vi "Get EventName.vi"(8 "error in (no error)":errorcluster, 11 "EventData in":refnum<class "EventData.lvclass">) -> (0 "error out":errorcluster, 2 "Event Name":string, 3 "EventData out":refnum<class "EventData.lvclass">)   [LabVIEW 2021, in "EventManagerLibrary.lvlib" / "EventData.lvclass"]
uses:
  EventData.lvclass
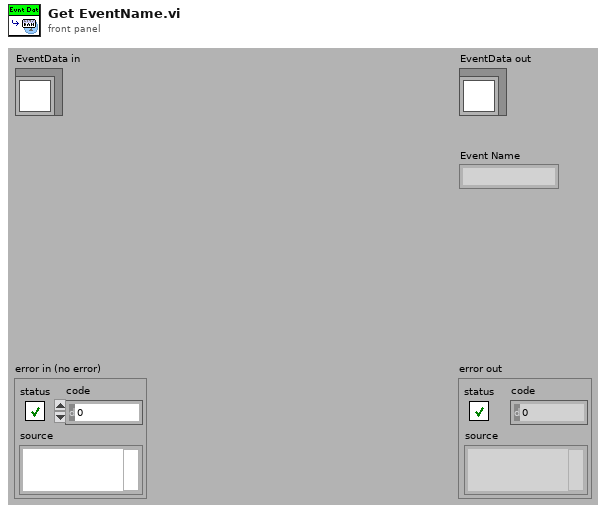
[diagram p1: front panel]
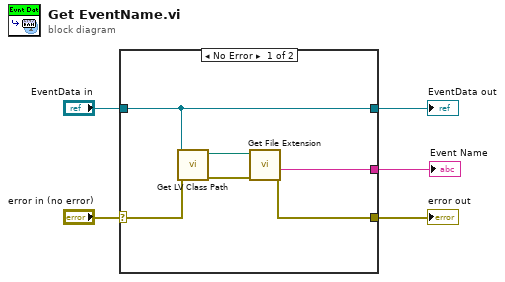
[diagram p0: block diagram]
diagram:
  n1 = case shown="No Error" "error in (no error)" {
    selector: "error in (no error)" -> [w8 w13]
    tunnel: [w7 w13] -> w2
    tunnel: [w11 w12] -> w4
    tunnel: "EventData in" -> [w11 w12]
    tunnel: [w6 _] -> w1
    frame No Error {
      n2 = call <vilib>:"Get LV Class Path.vi"("error in (no error)"=w8, "object"=w11) -> ("error out"=w9:errorcluster, "class path"=w10:path)  [unwired: 8 out]
      n3 = call <vilib>:"Get File Extension.vi"("error in (no error)"=w9, "file"=w10) -> ("error out"=w7:errorcluster, "filename without extension"=w6:string)  [unwired: 8 out]
    }
    frame Error {
    }
  }
  "error out" <- w2
  "EventData out" <- w4
  "Event Name" <- w1
